vi "InitLanguageSettings.vi"() -> ()   [LabVIEW 2013]
uses:
  <vilib>/Utility/config.llb/Read Key (String).vi
  GlobalVariables/LanguagesSettings.vi
  <vilib>/Utility/config.llb/NI_LVConfig.lvlib
panel:
  in  "error in":errorcluster
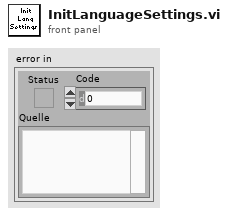
[diagram p1: front panel]
types:
  T1 = typedef "NI_LVConfig.lvlib/Config Data RefNum.ctl" = refnum<k1>
  T2 = cluster{"Indices":u32[], "LocalizedWords":string[][]}
  T3 = cluster{"Slices":string[], "value":string, i32, "LocalisationFileContent[out]":cluster{"Indices":u32[], "LocalizedWords":string[][]}}
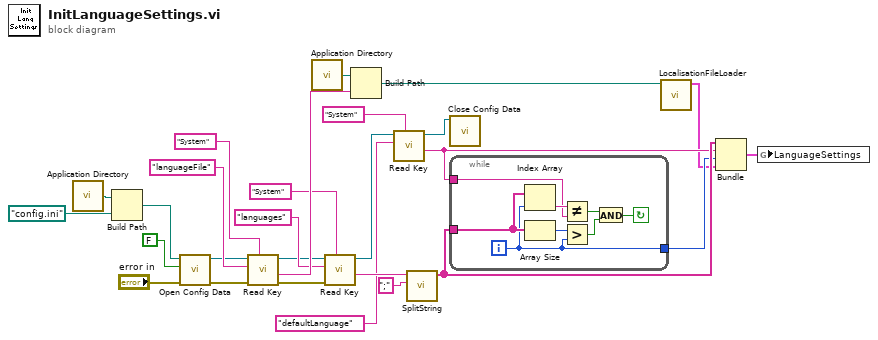
[diagram p0: block diagram]
diagram:
  n1 = call <vilib>:"Application Directory.vi"() -> ("Application Directory"=w21:path)
  n2 = Build Path(base path=w21, name or relative path=path "config.ini" ("default name")) -> (appended path=w25:path)
  n3 = call <vilib>:"Open Config Data.vi"("error in (no error)"="error in", "create file if necessary (T)"=FALSE ("create file if necessary? (T)"), "configuration file path"=w25) -> ("error out"=w24:errorcluster, "refnum"=w22:T1)  [unwired: 6 in, 1 out]
  n4 = call-poly <vilib>:"Read Key.vi"("section"="System", "error in (no error)"=w24, "key"="languageFile", "refnum"=w22) -> ("error out"=w13:errorcluster, "value"=w17:string, "refnum out"=w12:T1)  [unwired: 4 in, 1 out]
  n5 = call <vilib>:"Application Directory.vi"() -> ("Application Directory"=w18:path)
  n6 = call-poly <vilib>:"Read Key.vi"("section"="System", "error in (no error)"=w13, "key"="languages", "refnum"=w12) -> ("value"=w11:string, "refnum out"=w9:T1)  [unwired: 4 in, 2 out]
  n7 = Build Path(base path=w18, name or relative path=w17) -> (appended path=w2:path)
  n8 = call-poly <vilib>:"Read Key.vi"("section"="System", "key"="defaultLanguage", "refnum"=w9) -> ("value"=w4:string, "refnum out"=w8:T1)  [unwired: 5 in, 2 out]
  n9 = call "SplitString.vi"("Separator"=";", "String[in]"=w11) -> ("Slices"=w5:string[])  [unwired: 9 in]
  n10 = call <vilib>:"Close Config Data.vi"("refnum"=w8) -> ()  [unwired: 9 in, 2 out]
  n11 = while {
    tunnel: w5 -> [w30]
    tunnel: w4 -> [w29]
    tunnel: [w28] -> w3
    i -> [w28]
    stop <- w35 continue-if-true
    n12 = Index Array(array=w30, index=w28) -> (element=w31:string)
    n13 = Array Size(array=w30) -> (size(s)=w33:i32)
    n14 = Not Equal?(x=w31, y=w29) -> (x != y?=w32:bool)
    n15 = Greater?(x=w33, y=w28) -> (0:w34:bool)
    n16 = And(x=w32, y=w34) -> (x .and. y?=w35:bool)
  }
  n17 = call "LocalisationFileLoader.vi"("FilePath"=w2) -> ("LocalisationFileContent[out]"=w1:T2)  [unwired: 10 in]
  n18 = Bundle("Slices"=w5, "value"=w4, w3, "LocalisationFileContent[out]"=w1) -> (w16:T3)  [unwired: 1 in]
  n19 = global write "LanguagesSettings.vi" "LanguageSettings"(w16) -> ()
